vi "getOutputRange.vi"(8 "error in (no error)":errorcluster, 11 "PressureServoActuatorClosed in":refnum<class "PressureServoActuatorClosed.lvclass">) -> (0 "error out":errorcluster, 2 "output range":cluster{"output high":dbl, "output low":dbl}={"output high"=100.0, "output low"=-100.0}, 3 "PressureServoActuatorClosed out":refnum<class "PressureServoActuatorClosed.lvclass">)   [LabVIEW 2015, in "PressureServoActuatorClosed.lvclass"]
uses:
  PressureServoActuatorClosed.lvclass
  PressureServoActuatorClosed.lvclass/PressureServoActuatorClosed.ctl
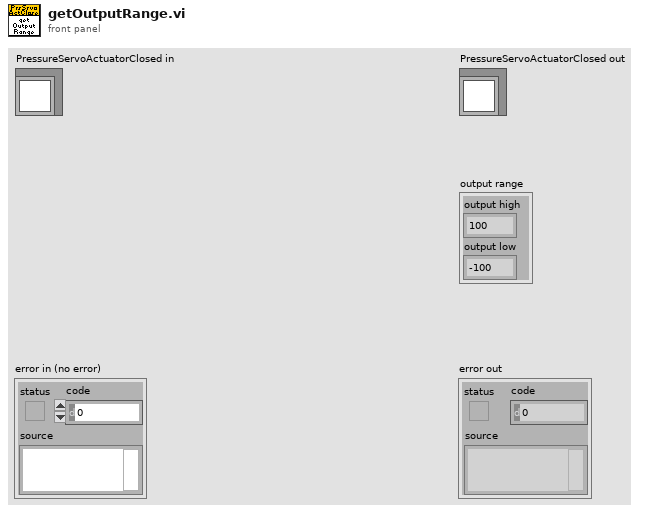
[diagram p1: front panel]
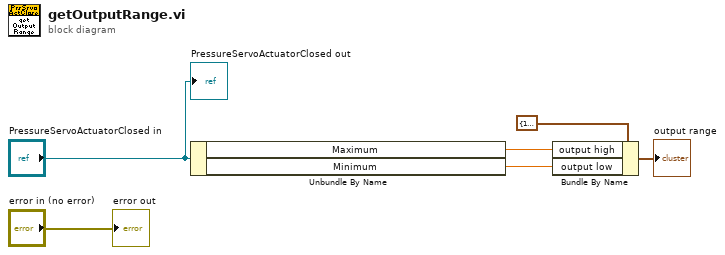
[diagram p0: block diagram]
diagram:
  n1 = Unbundle By Name("PressureServoActuatorClosed in") -> ("Maximum"=w2:dbl, "Minimum"=w1:dbl)
  n2 = Bundle By Name(cluster=cluster{"output high":dbl, "output low":dbl} {"output high"=100.0, "output low"=-100.0} ("output range"), "output high"=w2, "output low"=w1) -> (→"output range":cluster{"output high":dbl, "output low":dbl})
  "error out" <- "error in (no error)"
  "PressureServoActuatorClosed out" <- "PressureServoActuatorClosed in"
